vi "time seperation from  date and time.vi"(11 "time and date":string[](array[string])) -> (3 "time array":string[](array[string]))   [LabVIEW 2017]
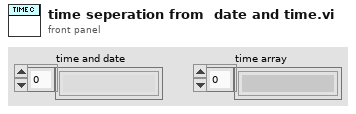
[diagram p1: front panel]
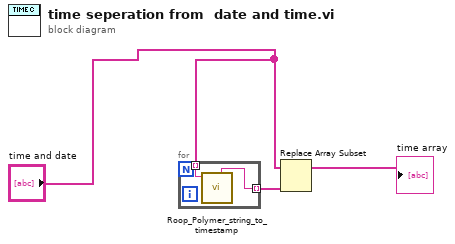
[diagram p0: block diagram]
diagram:
  n1 = for {
    tunnel: [w5] -> w1 mode=indexing
    tunnel: "time and date" -> [w4] mode=indexing
    n2 = call "Roop_Polymer_string_to_timestamp.vi"("String"=w4) -> ("time"=w5:string)  [unwired: 8 in, 2 out]
  }
  n3 = Replace Array Subset(array="time and date", new element=w1) -> (→"time array":string[])  [unwired: 1 in]
